vi "fg_path.vi"(8 "error in (no error)":errorcluster, 11 "custom_path":path) -> (0 "error out":errorcluster, 3 "config_working":path)   [LabVIEW 2015, in "lv-config-json.lvlib"]
doc: "Returns the location for the configuration, if provided a custom path, it will pass that path through."
uses:
  lv-config-json.lvlib
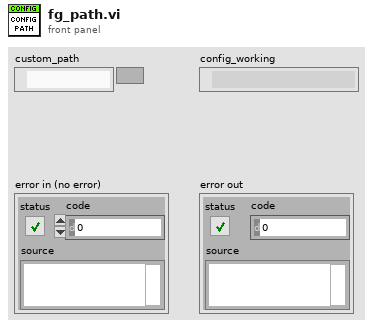
[diagram p1: front panel]
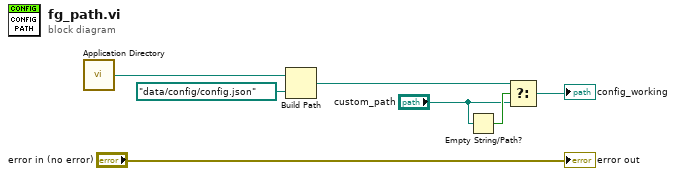
[diagram p0: block diagram]
diagram:
  n1 = call <vilib>:"Application Directory.vi"() -> ("Application Directory"=w6:path)
  n2 = Build Path(base path=w6, name or relative path=path "data/config/config.json" ("Application Directory")) -> (appended path=w2:path)
  n3 = Empty String/Path?(string/path="custom_path") -> (empty?=w4:bool)
  n4 = Select(t=w2, s=w4, f="custom_path") -> (s? t:f=→"config_working":path)
  "error out" <- "error in (no error)"
